vi "Dual DC Voltmeter.vi"() -> ()   [LabVIEW 2009]
uses:
  <vilib>/DAQmx/read.llb/DAQmx Read (Analog 2D DBL NChan NSamp).vi
  <vilib>/DAQmx/configure/timing.llb/DAQmx Timing (Sample Clock).vi
  <vilib>/DAQmx/create/channels.llb/DAQmx Create Channel (AI-Voltage-Basic).vi
  <vilib>/Analysis/NI_AALBase.lvlib
panel:
  in  "Input Voltage C":tag
  out "Voltage C":dbl[](graph)
  out "Mean Voltage Channel C":dbl format="%#.4f"
  out "Voltage B":dbl[](graph)
  out "Voltage A":dbl[](graph)
  in  "?":bool
  out "Mean Voltage Channel B":dbl format="%#.4f"
  out "Mean Voltage Channel A":dbl format="%#.4f"
  in  "Input Voltage B":tag
  in  "Input Voltage A":tag
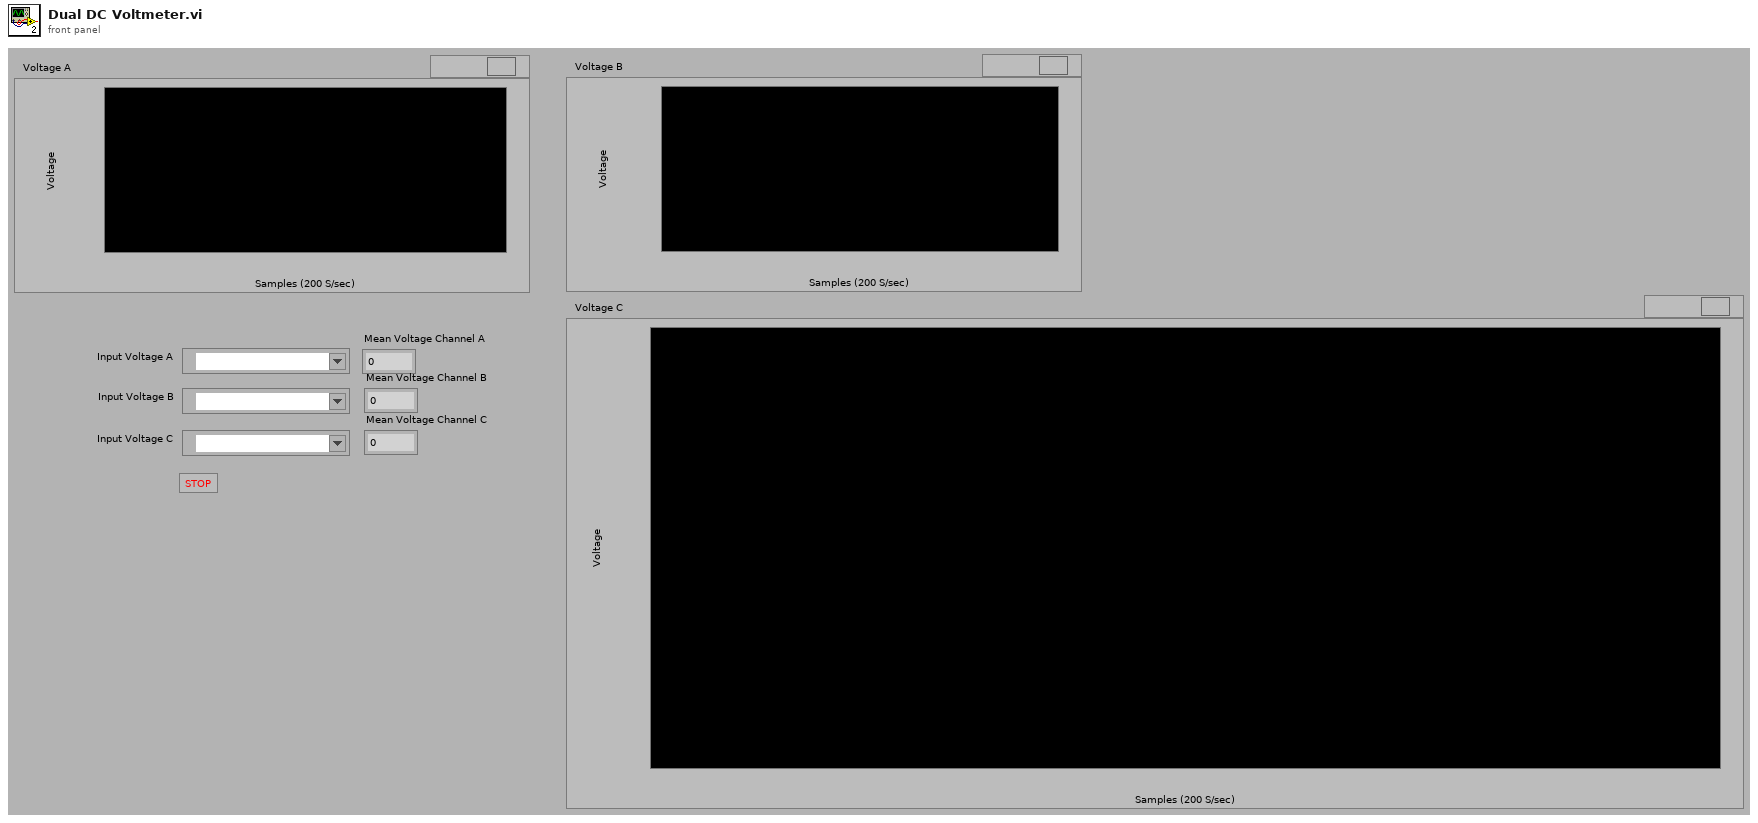
[diagram p1: front panel]
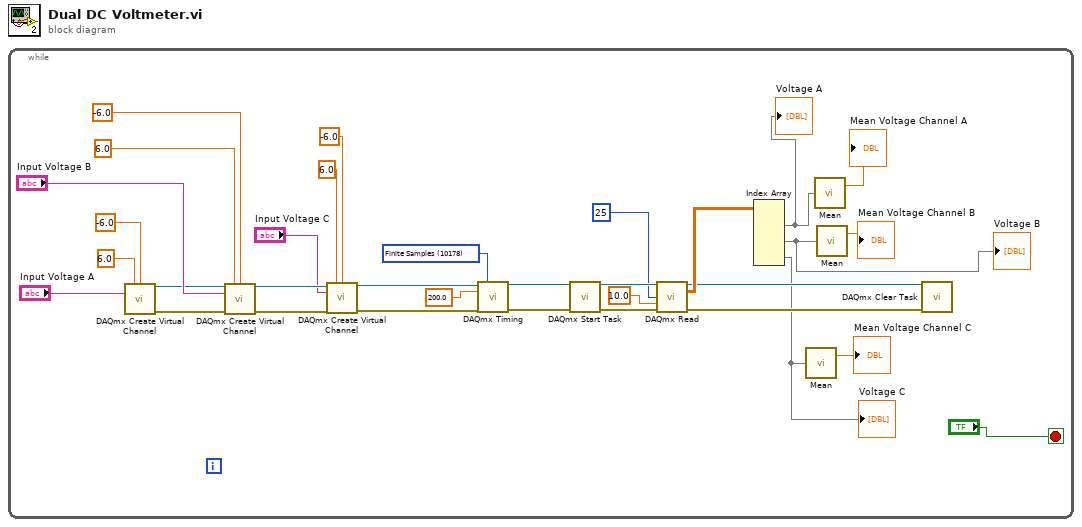
[diagram p0: block diagram]
diagram:
  n1 = while {
    stop <- "?" stop-if-true
    w25 = 10178 items=["Finite Samples"=10178, "Continuous Samples"=10123, "Hardware Timed Single Point"=12522] ("sample mode")
    n2 = call-poly <vilib>:"DAQmx Create Virtual Channel.vi"("maximum value"=6.0, "minimum value"=-6.0 ("maximum value"), "physical channels"="Input Voltage A") -> ("task out"=w27:refnum<k21>, "error out"=w26:errorcluster)  [unwired: 6 in, 5 out]
    n3 = call-poly <vilib>:"DAQmx Create Virtual Channel.vi"("task in"=w27, "maximum value"=6.0, "minimum value"=-6.0 ("maximum value"), "physical channels"="Input Voltage B", "error in"=w26) -> ("task out"=w9:refnum<k21>, "error out"=w8:errorcluster)  [unwired: 4 in, 5 out]
    n4 = call-poly <vilib>:"DAQmx Create Virtual Channel.vi"("task in"=w9, "maximum value"=6.0, "minimum value"=-6.0 ("maximum value"), "physical channels"="Input Voltage C", "error in"=w8) -> ("task out"=w6:refnum<k21>, "error out"=w7:errorcluster)  [unwired: 4 in, 5 out]
    n5 = call-poly <vilib>:"DAQmx Timing.vi"("task/channels in"=w6, "sample mode"=w25, "rate"=200.0, "error in"=w7) -> ("task out"=w24:refnum<k21>, "error out"=w23:errorcluster)  [unwired: 3 in, 7 out]
    n6 = call <vilib>:"DAQmx Start Task.vi"("task/channels in"=w24, "error in"=w23) -> ("task out"=w22:refnum<k21>, "error out"=w21:errorcluster)  [unwired: 12 out]
    n7 = call-poly <vilib>:"DAQmx Read.vi"("task/channels in"=w22, "number of samples per channel"=25, "timeout"=10.0, "error in"=w21) -> ("task out"=w16:refnum<k21>, "data"=w19:dbl[][], "error out"=w15:errorcluster)  [unwired: 9 out]
    n8 = Index Array(array=w19) -> (element #1=w13:dbl[], element #2=w12:dbl[], element #3=w2:dbl[])  [unwired: 6 in]
    "Voltage A" <- w13
    "Voltage B" <- w12
    "Voltage C" <- w2
    n9 = call <vilib>:"Mean.vi"("X"=w2) -> ("mean"=→"Mean Voltage Channel C":dbl)  [unwired: 1 out]
    n10 = call <vilib>:"Mean.vi"("X"=w13) -> ("mean"=→"Mean Voltage Channel A":dbl)  [unwired: 1 out]
    n11 = call <vilib>:"Mean.vi"("X"=w12) -> ("mean"=→"Mean Voltage Channel B":dbl)  [unwired: 1 out]
    n12 = call <vilib>:"DAQmx Clear Task.vi"("task in"=w16, "error in"=w15) -> ()  [unwired: 14 out]
  }
